vi "CleanDependencies.vi"(8 "error in (no error)":errorcluster, 10 "Dependency":refnum<class "SMO.lvclass">, 11 "SMO in":refnum<class "SMO.lvclass">) -> (0 "error out":errorcluster, 3 "SMO out":refnum<class "SMO.lvclass">, 4 "Removed":bool)   [LabVIEW 2019, in "SMO.lvclass"]
doc: "JKI State Machine Objects (SMO) 1.3.0.56\nJKI - JKI\nCopyright (c) 2017, JKI"
uses:
  SMO.lvclass
  SMO.lvclass/SMO.ctl
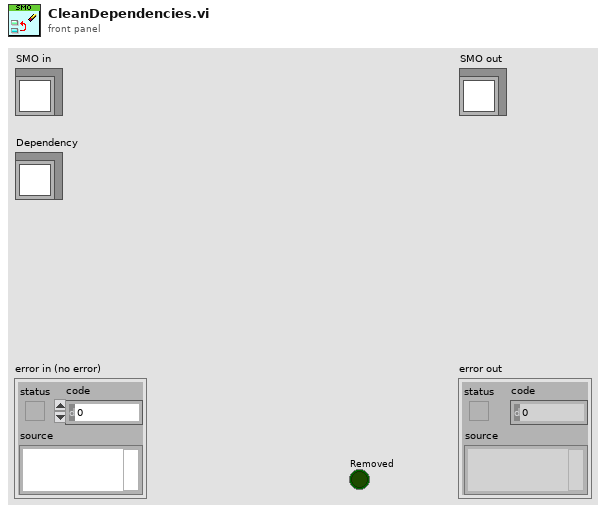
[diagram p1: front panel]
types:
  T1 = typedef "SMO.lvclass/PrivateData--Ref.ctl" = refnum<data-value>
  T2 = typedef "SMO.lvclass/PrivateData--Cluster.ctl" = cluster{"Parent Call":T3, "Registered Processes":T4[], "Sync Notifier":refnum<notifier>, "Process Error Notifier":refnum<notifier>, "Protected Events":T5, "Public Events":T6, "SMO State":T7, "[Dependencies]":T8[], "[Attributes]":refnum<class "Attribute.lvclass">[], "Launcher Close":refnum<notifier>, "Caller Watchdog":refnum<queue>, "Accessibility":T9, "NbStaticDependencies":u32}
  T3 = typedef "SMO.lvclass/Parent Call--Enum.ctl" = enum16{"Allows parent to run", "Does not request parent to run"}
  T4 = typedef "SMO.lvclass/RegisteredProcessData--Cluster.ctl" = cluster{"Name":string, "Static VI Ref":refnum<vi>, "Running":bool, "NotifierRef":u32}
  T5 = typedef "SMO.lvclass/Protected Events.ctl" = cluster{"StopProcesses":refnum<user-event>, "AbortProcesses":refnum<user-event>, "Config Changed":refnum<user-event>, "Dependency":refnum<user-event>}
  T6 = typedef "SMO.lvclass/Public Events.ctl" = cluster{"Error":refnum<user-event>, "State":refnum<user-event>, "Reserve State":refnum<user-event>}
  T7 = typedef "SMO.lvclass/SMOState --Enum.ctl" = enum16{"unknown", "Created", "Started", "Stopped"}
  T8 = typedef "SMO.lvclass/SMO Dependency--Cluster.ctl" = cluster{"Dependency":refnum<class "SMO.lvclass">, "Level":string}
  T9 = typedef "SMO.lvclass/Accessibility--Cluster.ctl" = cluster{"Lock Key":string, "Reserve State":T10}
  T10 = typedef "SMO.lvclass/Reserve State--Enum.ctl" = enum16{"Unreserved", "Reserved", "Self-locked"}
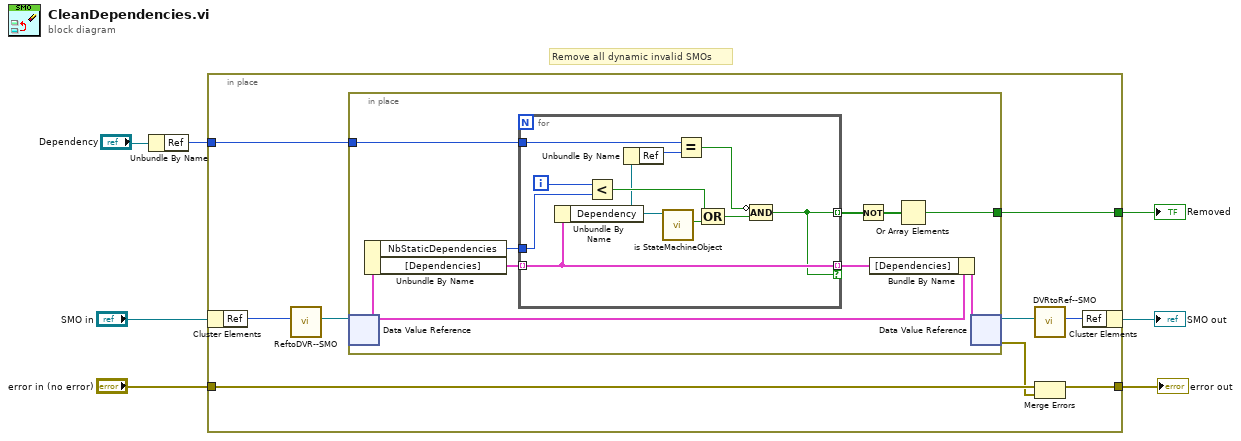
[diagram p0: block diagram]
diagram:
  # "Remove all dynamic invalid SMOs"
  n1 = Unbundle By Name("Dependency") -> ("Ref"=w1:u32)
  n2 = in-place {
    in-place-border: "error in (no error)" -> [w13]
    in-place-border: [w11] -> w6
    in-place-border: [w9] -> w3
    in-place-border: w1 -> [w8]
    n3 = in-place-cluster #1("SMO in") -> ("Ref"=w10:u32)
    n4 = call "ReftoDVR--SMO.vi"("Ref"=w10) -> ("Ref"=w16:T1)  [unwired: 10 in]
    n5 = in-place {
      in-place-border: [w19] -> w9
      in-place-border: w8 -> [w18]
      n6 = in-place-dvr #2(w16) -> (w25:T2)  [unwired: 1 out]
      n7 = Unbundle By Name(w25) -> ("NbStaticDependencies"=w17:u32, "[Dependencies]"=w23:T8[])
      n8 = for {
        tunnel: w23 -> [w36] mode=indexing
        tunnel: [w36] -> w22 mode=indexing if=w27
        tunnel: [w27] -> w21 mode=indexing
        tunnel: w18 -> [w31]
        tunnel: w17 -> [w26]
        i -> [w35]
        n9 = Unbundle By Name(w36) -> ("Dependency"=w32:refnum<class "SMO.lvclass">)
        n10 = Less?(x=w35, y=w26) -> (x < y?=w33:bool)
        n11 = Unbundle By Name(w32) -> ("Ref"=w30:u32)
        n12 = call "is StateMachineObject.vi"("SMO"=w32) -> ("is SMO?"=w34:bool)  [unwired: 8 in, 2 out]
        n13 = Equal?(x=w31, y=w30) -> (x = y?=w29:bool)
        n14 = Compound Arithmetic op=OR(w33, w34) -> (w28:bool)
        n15 = Compound Arithmetic op=AND(invert w29, w28) -> (w27:bool)
      }
      n16 = Not(x=w21) -> (.not. x?=w20:bool[])
      n17 = Bundle By Name(cluster=w25, "[Dependencies]"=w22) -> (w24:T2)
      n18 = Or Array Elements(Boolean array=w20) -> (logical OR=w19:bool)
      n19 = in-place-dvr #2(w24) -> (w15:T1, w12:errorcluster)
    }
    n20 = call "DVRtoRef--SMO.vi"("Ref"=w15) -> ("Ref"=w14:u32)  [unwired: 10 in]
    n21 = Merge Errors(w13, w12) -> (w11:errorcluster)
    n22 = in-place-cluster #1("Ref"=w14) -> (→"SMO out":refnum<class "SMO.lvclass">)
  }
  "error out" <- w6
  "Removed" <- w3
